vi "SMU Switch Handshaking - LV code improvements.vi"(8 "error in":errorcluster, 10 "Error Stream gRPCid":T1, 11 "file path (use dialog)":path=path "/home/lvuser/jsontestfile.json") -> (0 "error out":errorcluster, 1 "Results":T2[](array[typedef]), 3 "Elapsed Time":u32)   [LabVIEW 2019]
uses:
  VIs/MeasurementServer_FourProbeRawData.ctl
  VIs/MeasurementServer_ErrorOutData.ctl
  VIs/MeasurementServer_gRPCid.ctl
  <instrlib>/niDCPower/nidcpower.llb/niDCPower Send Software Edge Trigger - Signal.ctl
  Global Operations.ctl
  <instrlib>/niDCPower/nidcpower.llb/niDCPower Configure Software Edge Start Trigger.vi
  <instrlib>/niDCPower/nidcpower.llb/niDCPower Configure Software Edge Sequence Advance Trigger.vi
  VIs/labview-grpc-measurement-server.lvlib
  SupportVIs.lvlib
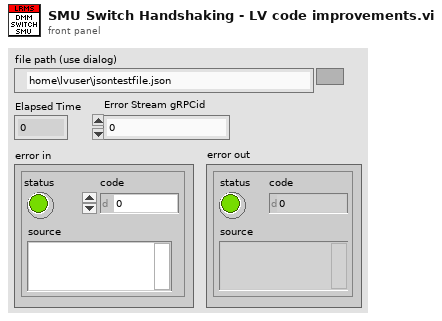
[diagram p1: front panel]
types:
  T1 = typedef "labview-grpc-measurement-server.lvlib/MeasurementServer_gRPCid.ctl" = u64
  T2 = typedef "labview-grpc-measurement-server.lvlib/MeasurementServer_FourProbeRawData.ctl" = cluster{"Positive Voltage":dbl, "Positive Current":dbl, "Negative Voltage":dbl, "Negative Current":dbl, "Impedance":dbl, "ErrorOutData":T3}
  T3 = typedef "labview-grpc-measurement-server.lvlib/MeasurementServer_ErrorOutData.ctl" = cluster{"ErrorCode":i32, "ErrorMessage":string}
  T4 = typedef "niDCPower Send Software Edge Trigger - Signal.ctl" = i32
  T5 = typedef "JSONCluster.ctl" = cluster{"SMUResourceName":string, "SMUChannels":string, "SMUSourceMode":i32, "SMUOutputFunction":i32, "SMUSourceTransientResponse":i32, "SMUCurrent":dbl, "SMUCurrentLevelRange":dbl, "SMUMeasurementSense":i32, "SMUMeasurementApertureTime":dbl, "SMUSourceAdvancedSourceDelay":dbl, "SMUVoltage":dbl, "SMUSourceAdvancedSequenceLoopCount":i32, "SMUMeasurementAdvancedDCNoiseRejection":i32, "SMUSequenceName":string, "SMUStep1_Source_DCCurrent_CurrentLevel":i32, "SMUStep2_Measurement_ApertureTime":i32, "SMUStep3_Source_Advanced_SourceDelay":i32, "SMUSequenceNumberOfSteps":i32, "ScanList":string, "Switch1ResourceName":string, "Switch1Topology":string, "Switch1ScanList":string, "Switch2ResourceName":string, "Switch2Topology":string, "Switch2ScanList":string, "DMMResourceName":string, "DMMFunction":i32, "DMMResolution":dbl, "DMMRange":dbl, "DMMSampleCount":i32, "DMMApertureTimeUnit":i32, "DMMApertureTime":dbl, "DMMNumberOfAverages":i32, "DMMAutoZero":i32, "DMMADCCalibration":i32, "DMMSettleTime":dbl, "DMMControlAction":i32, "DMMVoltageFaultUpperLimit":dbl, "ApplicationNumberOfWeldChannels":i32}
  T6 = typedef "Global Operations.ctl" = enum16{"Get", "Set"}
  T7 = typedef "niDMM Acquisition State.ctl" = enum16{"Running", "Finished with Backlog", "Finished with no Backlog", "Paused", "No acquisition in progress"}
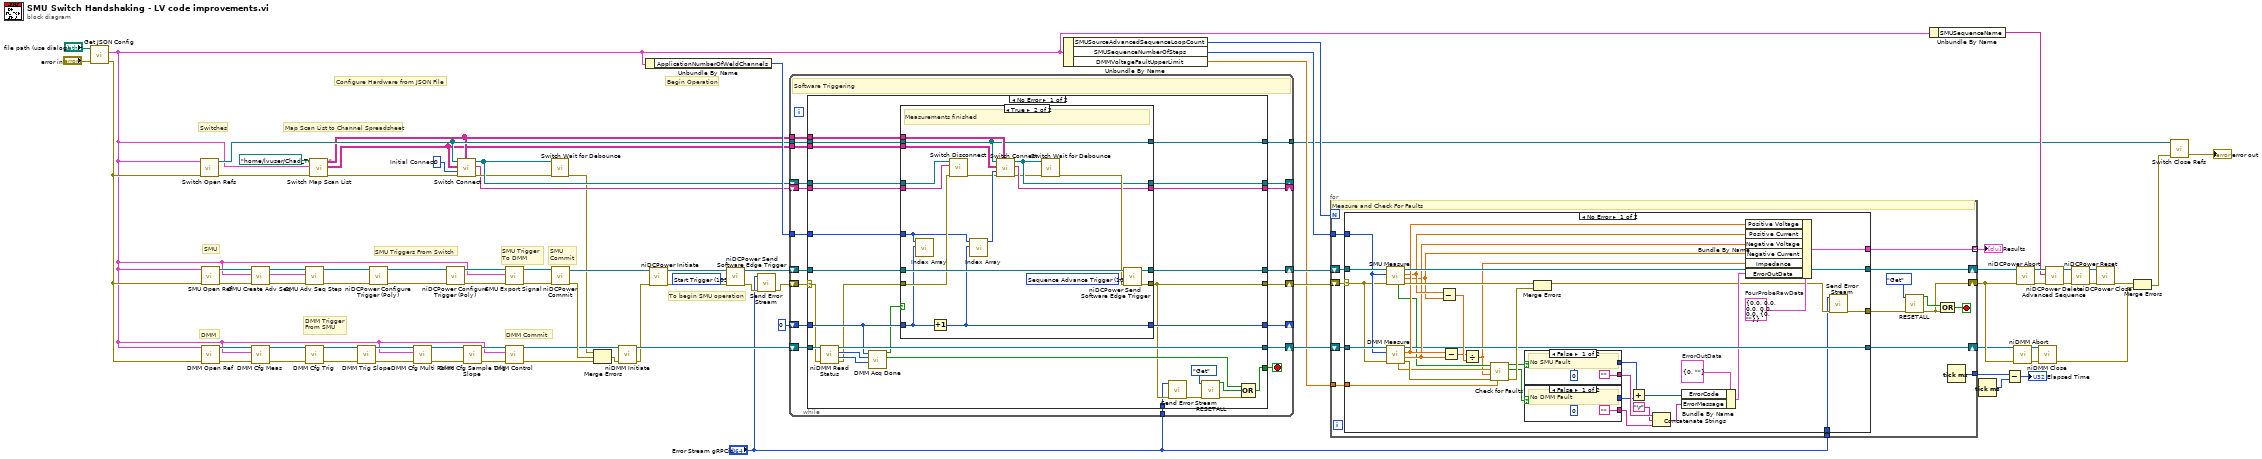
[diagram p0: block diagram]
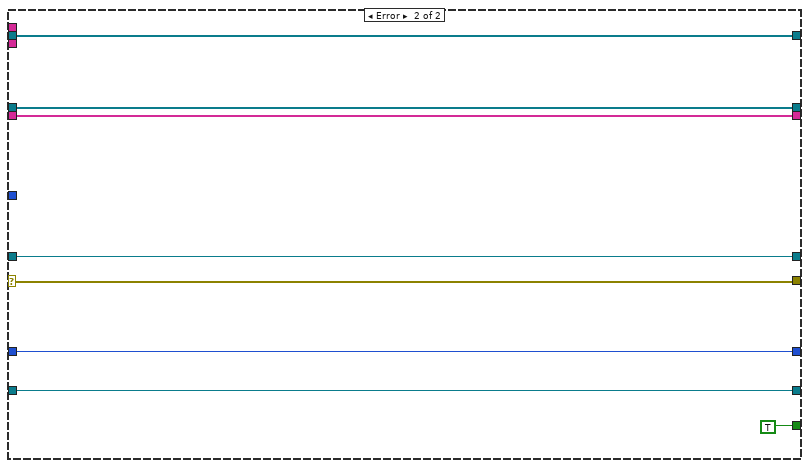
[diagram p3: hidden frame]
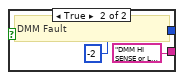
[diagram p4: hidden frame]
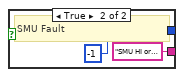
[diagram p5: hidden frame]
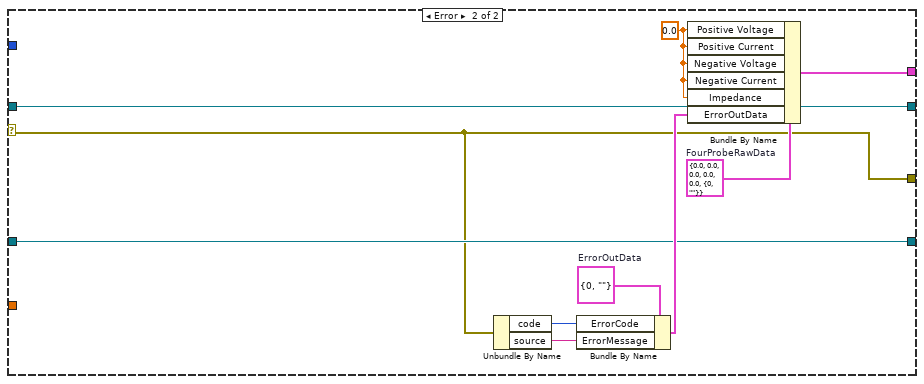
[diagram p6: hidden frame]
diagram:
  w4 = 0  # Initial Connect
  w30 = T4 1034 items=["Start Trigger"=1034, "Source Trigger"=1035, "Measure Trigger"=1036, "Sequence Advance Trigger"=1037, "Pulse Trigger"=1053] ("signal")
  # "Map Scan List to Channel Spreadsheet"
  # "SMU\nCommit"
  # "DMM Commit"
  # "Begin Operation"
  # "Configure Hardware from JSON File"
  # "DMM"
  # "SMU"
  # "Switches"
  # "To begin SMU operation"
  # "DMM Trigger\nFrom SMU"
  # "SMU Trigger \nTo DMM"
  # "SMU Triggers From Switch"
  n1 = call "Get JSON Config.vi"("error in (no error)"="error in", "JSON Configuration File (.json)"="file path (use dialog)") -> ("error out"=w18:errorcluster, "JSONCluster"=w1:T5)  [unwired: 6 in, 2 out]
  n2 = call "Switch Open Refs.vi"("error in (no error)"=w18, "JSONCluster"=w1) -> ("error out"=w7:errorcluster, "Switch Refs"=w12:refnum<k15>[])  [unwired: 8 in]
  n3 = call "SMU Open Ref.vi"("error in (no error)"=w18, "JSONCluster"=w1) -> ("error out"=w81:errorcluster, "IVI Refnum out"=w82:refnum<k15>)  [unwired: 8 in]
  n4 = call "DMM Open Ref.vi"("error in"=w18, "JSONCluster"=w1) -> ("error out"=w54:errorcluster, "IVI Refnum out"=w53:refnum<k15>)  [unwired: 8 in]
  n5 = call "SMU Create Adv Seq.vi"("error in (no error)"=w81, "JSONCluster"=w1, "IVI Refnum in"=w82) -> ("error out"=w69:errorcluster, "IVI Refnum out"=w70:refnum<k15>)  [unwired: 7 in]
  n6 = call "DMM Cfg Meas.vi"("error in (no error)"=w54, "JSONCluster"=w1, "IVI Refnum in"=w53) -> ("error out"=w58:errorcluster, "IVI Refnum out"=w57:refnum<k15>)  [unwired: 7 in]
  n7 = call "SMU Adv Seq Step.vi"("error in (no error)"=w69, "JSONCluster"=w1, "IVI Refnum in"=w70) -> ("error out"=w67:errorcluster, "IVI Refnum out"=w68:refnum<k15>)  [unwired: 7 in]
  n8 = call "DMM Cfg Trig.vi"("error in (no error)"=w58, "IVI Refnum in"=w57) -> ("error out"=w60:errorcluster, "IVI Refnum out"=w59:refnum<k15>)  [unwired: 8 in]
  n9 = call "Switch Map Scan List.vi"("error in (no error)"=w7, "JSONCluster"=w1, "Ch Spreadsheet"=path "/home/lvuser/Chad_Test.csv") -> ("error out"=w6:errorcluster, "IVI Specifications"=w10:string[][], "Channel Specs"=w11:string[][])  [unwired: 6 in]
  n10 = call "DMM Trig Slope.vi"("error in (no error)"=w60, "IVI Refnum in"=w59) -> ("error out"=w62:errorcluster, "IVI Refnum out"=w61:refnum<k15>)  [unwired: 8 in]
  n11 = call-poly <instrlib>:"niDCPower Configure Trigger (Poly).vi"("error in (no error)"=w67, "instrument handle"=w68) -> ("error out"=w78:errorcluster, "instrument handle out"=w79:refnum<k15>)  [unwired: 8 in]
  n12 = call "DMM Cfg Multi Point.vi"("error in (no error)"=w62, "JSONCluster"=w1, "IVI Refnum in"=w61) -> ("error out"=w64:errorcluster, "IVI Refnum out"=w63:refnum<k15>)  [unwired: 7 in]
  n13 = call-poly <instrlib>:"niDCPower Configure Trigger (Poly).vi"("error in (no error)"=w78, "instrument handle"=w79) -> ("error out"=w40:errorcluster, "instrument handle out"=w41:refnum<k15>)  [unwired: 8 in]
  n14 = call "Switch Connect.vi"("Channel Specs"=w11, "error in (no error)"=w6, "Channel Index"=w4, "IVI Specifications"=w10, "Switch Refs"=w12) -> ("error out"=w5:errorcluster, "Channels Connected"=w3:string[], "Refs Connected"=w13:refnum<k15>[])  [unwired: 4 in]
  n15 = call "DMM Cfg Sample Trig Slope.vi"("error in (no error)"=w64, "IVI Refnum in"=w63) -> ("error out"=w46:errorcluster, "IVI Refnum out"=w47:refnum<k15>)  [unwired: 8 in]
  n16 = call "SMU Export Signal.vi"("error in (no error)"=w40, "JSONCluster"=w1, "IVI Refnum in"=w41) -> ("error out"=w65:errorcluster, "IVI Refnum out"=w66:refnum<k15>)  [unwired: 7 in]
  n17 = call "DMM Control.vi"("error in (no error)"=w46, "JSONCluster"=w1, "IVI Refnum in"=w47) -> ("error out"=w51:errorcluster, "IVI Refnum out"=w48:refnum<k15>)  [unwired: 7 in]
  n18 = call "Switch Wait for Debounce.vi"("error in (no error)"=w5, "Switch Refs"=w13) -> ("error out"=w2:errorcluster)  [unwired: 9 in]
  n19 = call <instrlib>:"niDCPower Commit.vi"("error in (no error)"=w65, "instrument handle"=w66) -> ("error out"=w52:errorcluster, "instrument handle out"=w49:refnum<k15>)  [unwired: 8 in]
  n20 = Merge Errors(w2, w52, w51) -> (w50:errorcluster)
  n21 = call <instrlib>:"niDMM Initiate.vi"("error in (no error)"=w50, "instrument handle"=w48) -> ("error out"=w23:errorcluster, "instrument handle out"=w29:refnum<k15>)  [unwired: 8 in]
  n22 = Unbundle By Name(w1) -> ("ApplicationNumberOfWeldChannels"=w25:i32)
  n23 = call <instrlib>:"niDCPower Initiate.vi"("error in (no error)"=w23, "instrument handle"=w49) -> ("error out"=w24:errorcluster, "instrument handle out"=w32:refnum<k15>)  [unwired: 8 in]
  n24 = call <instrlib>:"niDCPower Send Software Edge Trigger.vi"("error in (no error)"=w24, "signal"=w30, "instrument handle"=w32) -> ("error out"=w16:errorcluster, "instrument handle out"=w31:refnum<k15>)  [unwired: 7 in]
  n25 = call "Send Error Stream.vi"("error in (no error)"=w16, "Error Stream gRPCid"="Error Stream gRPCid") -> ("error out"=w15:errorcluster)  [unwired: 9 in]
  n26 = while {
    shift-right: [w101] -> w34
    shift-left: w31 -> [w98]
    shift-right: [w99] -> w33
    shift-left: w15 -> [w92]
    shift-right: [w96] -> w28
    shift-left: w29 -> [w97]
    shift-right: [w94] -> _
    shift-left: 0 ("Backlog") -> [w95]
    tunnel: w25 -> [w93]
    tunnel: "Error Stream gRPCid" -> [w91]
    shift-right: [w87] -> _
    shift-left: w13 -> [w89]
    shift-right: [w86] -> _
    shift-left: w3 -> [w90]
    tunnel: w12 -> [w88]
    tunnel: w11 -> [w85]
    tunnel: w10 -> [w84]
    tunnel: [w83] -> w9
    stop <- w100 stop-if-true
    # "Software Triggering"
    n27 = case shown="No Error" w92 {
      selector: w92 -> [w118 w161]
      tunnel: [w129 w162] -> w101
      tunnel: [w113 TRUE] -> w100
      tunnel: [w112 w161] -> w99
      tunnel: w98 -> [w128 w162]
      tunnel: w97 -> [w125 w159]
      tunnel: [w124 w159] -> w96
      tunnel: w95 -> [w123 w160]
      tunnel: [w122 w160] -> w94
      tunnel: w93 -> [w120 _]
      tunnel: w91 -> [w111 _]
      tunnel: w90 -> [w108 w156]
      tunnel: w89 -> [w109 w157]
      tunnel: w88 -> [w107 w155]
      tunnel: [w106 w157] -> w87
      tunnel: [w105 w156] -> w86
      tunnel: w85 -> [w104 _]
      tunnel: w84 -> [w103 _]
      tunnel: [w102 w155] -> w83
      frame No Error {
        n28 = call <instrlib>:"niDMM Read Status.vi"("error in (no error)"=w118, "instrument handle"=w125) -> ("error out"=w119:errorcluster, "Acquisition State"=w127:T7, "Backlog"=w126:i32, "instrument handle out"=w124:refnum<k15>)  [unwired: 6 in]
        n29 = call "DMM Acq Done.vi"("Acquisition State"=w127, "Backlog"=w126, "Channel Index"=w123) -> ("Finished with Backlog?"=w114:bool, "Sequence Acquision Finished?"=w121:bool)  [unwired: 7 in]
        n30 = case shown="True" w121 {
          tunnel: w119 -> [w134 w150]
          tunnel: [w135 w154] -> w129
          tunnel: [w134 w153] -> w112
          tunnel: w128 -> [w135 w151]
          tunnel: w123 -> [w133 w148]
          tunnel: [w133 w146] -> w122
          tunnel: w120 -> [_ w145]
          tunnel: w109 -> [w132 w143]
          tunnel: w108 -> [w131 w144]
          tunnel: w107 -> [w130 w138]
          tunnel: [w132 w142] -> w106
          tunnel: [w131 w141] -> w105
          tunnel: w104 -> [_ w140]
          tunnel: w103 -> [_ w139]
          tunnel: [w130 w138] -> w102
          frame False {
            # "Measurements not finished yet - repeat loop"
          }
          frame True {
            w152 = T4 1037 items=["Start Trigger"=1034, "Source Trigger"=1035, "Measure Trigger"=1036, "Sequence Advance Trigger"=1037, "Pulse Trigger"=1053] ("signal")
            # "Measurements finished"
            n31 = call "Index Array.vi"("Backlog"=w148, "ApplicationNumberOfWeldChannels"=w145) -> ()  [unwired: 9 in, 1 out]
            n32 = Increment(x=w148) -> (x+1=w146:i32)
            n33 = call "Switch Disconnect.vi"("error in (no error)"=w150, "Channels Connected"=w144, "Switch Refs"=w143) -> ("error out"=w137:errorcluster)  [unwired: 8 in]
            n34 = call "Index Array.vi"("Backlog"=w146, "ApplicationNumberOfWeldChannels"=w145) -> ("Index"=w147:i32)  [unwired: 9 in]
            n35 = call "Switch Connect.vi"("Channel Specs"=w140, "error in (no error)"=w137, "Channel Index"=w147, "IVI Specifications"=w139, "Switch Refs"=w138) -> ("error out"=w136:errorcluster, "Channels Connected"=w141:string[], "Refs Connected"=w142:refnum<k15>[])  [unwired: 4 in]
            n36 = call "Switch Wait for Debounce.vi"("error in (no error)"=w136, "Switch Refs"=w142) -> ("error out"=w149:errorcluster)  [unwired: 9 in]
            n37 = call <instrlib>:"niDCPower Send Software Edge Trigger.vi"("error in (no error)"=w149, "signal"=w152, "instrument handle"=w151) -> ("error out"=w153:errorcluster, "instrument handle out"=w154:refnum<k15>)  [unwired: 7 in]
          }
        }
        n38 = call "Send Error Stream.vi"("error in (no error)"=w112, "Error Stream gRPCid"=w111) -> ("error out"=w110:errorcluster)  [unwired: 9 in]
        n39 = call "RESETALL.vi"("error in (no error)"=w110, "Operation"=Global_Operations."Get") -> ("error out"=w116:errorcluster, "RESETALL?"=w115:bool)  [unwired: 8 in]
        n40 = Compound Arithmetic op=OR(w114, w115, w116) -> (w113:bool)
      }
      frame Error {
      }
    }
  }
  n41 = Unbundle By Name(w1) -> ("SMUSourceAdvancedSequenceLoopCount"=w36:i32, "SMUSequenceNumberOfSteps"=w35:i32, "DMMVoltageFaultUpperLimit"=w17:dbl)
  n42 = for {
    N: w36 -> [_]
    tunnel: w35 -> [w174]
    shift-right: [w165] -> w45
    shift-left: w33 -> [w169]
    shift-right: [w177] -> w80
    shift-left: w34 -> [w175]
    shift-right: [w173] -> w42
    shift-left: w28 -> [w176]
    tunnel: [w172] -> w21 mode=indexing
    tunnel: [w171] -> w19
    tunnel: w17 -> [w170]
    tunnel: "Error Stream gRPCid" -> [w163]
    stop <- w166 stop-if-true
    # "Measure and Check For Faults"
    n43 = case shown="No Error" w169 {
      selector: w169 -> [w181 w221]
      tunnel: [w212 w223] -> w177
      tunnel: w176 -> [w211 w222]
      tunnel: w175 -> [w205 w223]
      tunnel: w174 -> [w204 _]
      tunnel: [w199 w222] -> w173
      tunnel: [w197 w225] -> w172
      tunnel: w170 -> [w182 _]
      tunnel: [w179 w221] -> w164
      tunnel: w163 -> [w178 _]
      frame No Error {
        w184 = T3 {"ErrorCode"=0, "ErrorMessage"=""}  # ErrorOutData
        w183 = T2 {"Positive Voltage"=0.0, "Positive Current"=0.0, "Negative Voltage"=0.0, "Negative Current"=0.0, "Impedance"=0.0, "ErrorOutData"={"ErrorCode"=0, "ErrorMessage"=""}}  # FourProbeRawData
        n44 = call "SMU Measure.vi"("error in (no error)"=w181, "SMUSequenceNumberOfSteps"=w204, "IVI Refnum in"=w205) -> ("error out"=w210:errorcluster, "Numeric"=w200:dbl, "Numeric 2"=w202:dbl, "IVI Refnum out"=w212:refnum<k15>, "in compliance"=w187:bool[])  [unwired: 4 in]
        n45 = call "DMM Measure.vi"("error in (no error)"=w181, "SMUSequenceNumberOfSteps"=w204, "IVI Refnum in"=w211) -> ("error out"=w209:errorcluster, "Numeric"=w201:dbl, "Numeric 2"=w203:dbl, "IVI Refnum out"=w199:refnum<k15>, "Measurements"=w186:dbl[])  [unwired: 4 in]
        n46 = Subtract(x=w202, y=w200) -> (x-y=w207:dbl)
        n47 = Subtract(x=w203, y=w201) -> (x-y=w206:dbl)
        n48 = Divide(x=w206, y=w207) -> (x/y=w185:dbl)
        n49 = call "Check for Faults.vi"("DMM Voltage Fault Upper Limit"=w182, "Error In"=w209, "Resistance In"=w185, "dmm voltage measurements"=w186, "in compliance"=w187) -> ("Error Out"=w208:errorcluster, "DMM Fault"=w191:bool, "SMU Fault"=w195:bool)  [unwired: 3 in, 1 out]
        n50 = case shown="False" w195 {
          tunnel: ["" "SMU HI or LO lead disconnected\n- SMU in compliance\n- SMU Fault = True"] -> w194
          tunnel: [0 -1] -> w192
          frame False {
            # "No SMU Fault"
          }
          frame True {
            # "SMU Fault"
          }
        }
        n51 = case shown="False" w191 {
          tunnel: ["" "DMM HI SENSE or LO SENSE lead disconnected\n- DMM measures NaN, or \n- DMM overrange warning, or\n- DMM voltage > 50uV "] -> w189
          tunnel: [0 -2] -> w188
          frame False {
            # "No DMM Fault"
          }
          frame True {
            # "DMM Fault"
          }
        }
        n52 = Merge Errors(w210, w208) -> (w180:errorcluster)
        n53 = Add(x=w192, y=w188) -> (x+y=w196:i32)
        n54 = Concatenate Strings(w194, "\r", w189) -> (w193:string)
        n55 = Bundle By Name(cluster=w184, "ErrorCode"=w196, "ErrorMessage"=w193) -> (w198:T3)
        n56 = Bundle By Name(cluster=w183, "Positive Voltage"=w203, "Positive Current"=w202, "Negative Voltage"=w201, "Negative Current"=w200, "Impedance"=w185, "ErrorOutData"=w198) -> (w197:T2)
        n57 = call "Send Error Stream.vi"("error in (no error)"=w180, "Error Stream gRPCid"=w178) -> ("error out"=w179:errorcluster)  [unwired: 9 in]
      }
      frame Error {
        w224 = 0.0 ("Positive Voltage")
        w228 = T3 {"ErrorCode"=0, "ErrorMessage"=""}  # ErrorOutData
        w229 = T2 {"Positive Voltage"=0.0, "Positive Current"=0.0, "Negative Voltage"=0.0, "Negative Current"=0.0, "Impedance"=0.0, "ErrorOutData"={"ErrorCode"=0, "ErrorMessage"=""}}  # FourProbeRawData
        n58 = Unbundle By Name(w221) -> ("code"=w226:i32, "source"=w227:string)
        n59 = Bundle By Name(cluster=w228, "ErrorCode"=w226, "ErrorMessage"=w227) -> (w230:T3)
        n60 = Bundle By Name(cluster=w229, "Positive Voltage"=w224, "Positive Current"=w224, "Negative Voltage"=w224, "Negative Current"=w224, "Impedance"=w224, "ErrorOutData"=w230) -> (w225:T2)
      }
    }
    n61 = call "RESETALL.vi"("error in (no error)"=w164, "Operation"=Global_Operations."Get") -> ("error out"=w165:errorcluster, "RESETALL?"=w167:bool)  [unwired: 8 in]
    n62 = Compound Arithmetic op=OR(w167, w165) -> (w166:bool)
    n63 = Tick Count (ms)() -> (millisecond timer value=w171:u32)
  }
  "Results" <- w21
  n64 = Unbundle By Name(w1) -> ("SMUSequenceName"=w20:string)
  n65 = Tick Count (ms)() -> (millisecond timer value=w77:u32)
  n66 = Subtract(x=w19, y=w77) -> (x-y=→"Elapsed Time":u32)
  n67 = call <instrlib>:"niDMM Abort.vi"("error in (no error)"=w45, "instrument handle"=w42) -> ("error out"=w56:errorcluster, "instrument handle out"=w55:refnum<k15>)  [unwired: 8 in]
  n68 = call <instrlib>:"niDCPower Abort.vi"("error in (no error)"=w45, "instrument handle"=w80) -> ("error out"=w75:errorcluster, "instrument handle out"=w76:refnum<k15>)  [unwired: 8 in]
  n69 = call <instrlib>:"niDMM Close.vi"("error in (no error)"=w56, "instrument handle"=w55) -> ("error out"=w44:errorcluster)  [unwired: 9 in]
  n70 = call <instrlib>:"niDCPower Delete Advanced Sequence.vi"("error in (no error)"=w75, "sequence name"=w20, "instrument handle"=w76) -> ("error out"=w74:errorcluster, "instrument handle out"=w73:refnum<k15>)  [unwired: 7 in]
  n71 = call <instrlib>:"niDCPower Reset.vi"("error in (no error)"=w74, "instrument handle"=w73) -> ("error out"=w71:errorcluster, "instrument handle out"=w72:refnum<k15>)  [unwired: 2 in, 6 out]
  n72 = call <instrlib>:"niDCPower Close.vi"("error in (no error)"=w71, "instrument handle"=w72) -> ("error out"=w43:errorcluster)  [unwired: 9 in]
  n73 = Merge Errors(w43, w44) -> (w26:errorcluster)
  n74 = call "Switch Close Refs.vi"("error in (no error)"=w26, "Switch Refs"=w9) -> ("error out"=→"error out":errorcluster)  [unwired: 9 in]
